vi "Test - copia (2).vi"() -> ()   [LabVIEW 2010]
panel:
  in  "Vi to open":enum16{"JILTest", "JILTest2", "JILTestR"}(ring)
  in  "stringin":string
  in  "booleanin":bool=TRUE
  in  "doublein":dbl
  in  "intin":i32
  in  "Mensajes":T1(ring)
  in  "stop":bool
  in  "Send":bool=TRUE
  out "error out":errorcluster
  out "Respuesta":string
  out "Mensaje":string
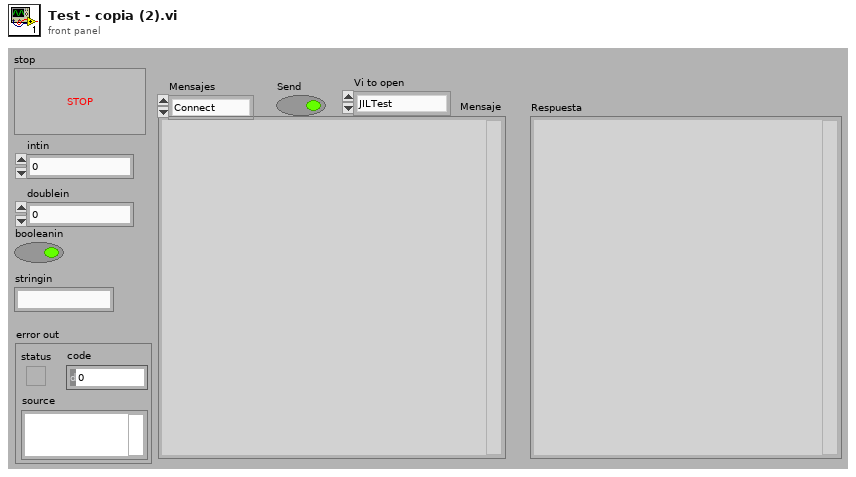
[diagram p1: front panel]
types:
  T1 = enum16{"Connect", "OpenVi", "SyncVi", "RunVi", "StopVi", "CloseVi", "Disconnect"}
  T2 = enum16{"Standard", "Buffered", "CRLF", "Immediate"}
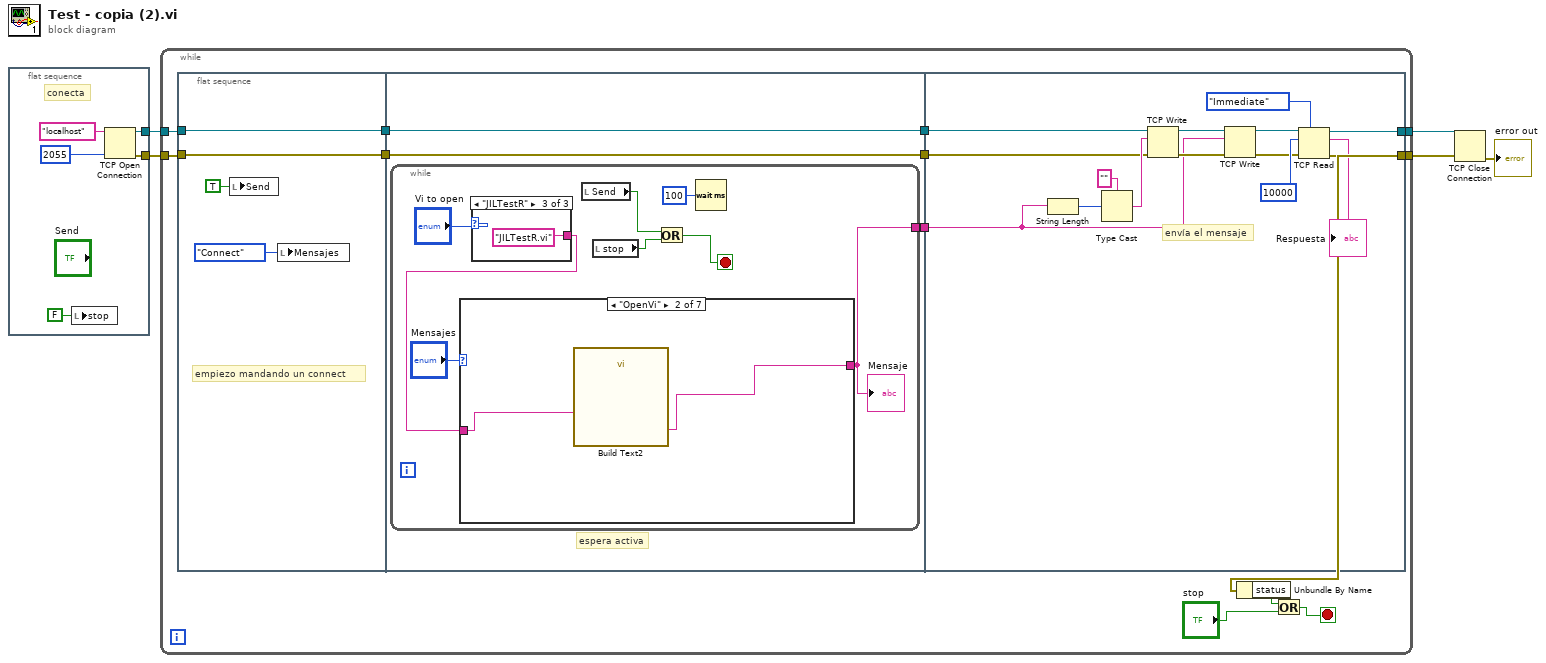
[diagram p0: block diagram]
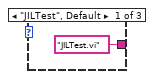
[diagram p2: hidden frame]
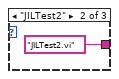
[diagram p3: hidden frame]
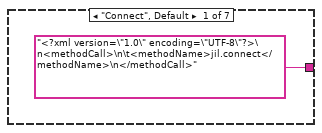
[diagram p4: hidden frame]
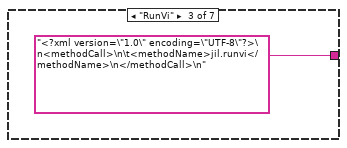
[diagram p5: hidden frame]
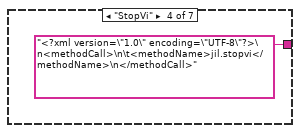
[diagram p6: hidden frame]
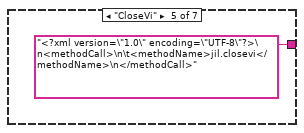
[diagram p7: hidden frame]
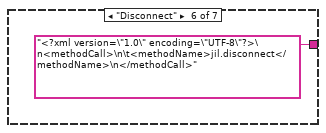
[diagram p8: hidden frame]
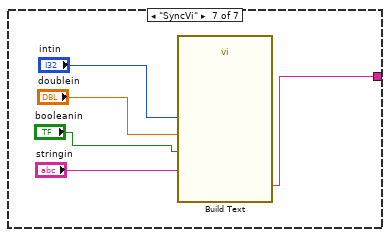
[diagram p9: hidden frame]
diagram:
  n1 = flat-sequence {
    tunnel: [w8] -> w5
    tunnel: [w7] -> w4
    frame #0 {
      # "conecta"
      n2 = local write "stop"(FALSE ("stop")) -> ()
      n3 = TCP Open Connection(address="localhost", remote port or service name=u16 2055) -> (connection ID=w8:refnum<k5>, error out=w7:errorcluster)  [unwired: 3 in]
    }
  }
  n4 = while {
    tunnel: w5 -> [w18]
    tunnel: w4 -> [w17]
    tunnel: [w16] -> w2
    tunnel: [w13] -> w1
    stop <- w14 stop-if-true
    n5 = flat-sequence {
      tunnel: w17 -> [w25]
      tunnel: [w25] -> w22
      tunnel: w18 -> [w24]
      tunnel: [w24] -> w21
      tunnel: w22 -> [w29]
      tunnel: [w29] -> w20
      tunnel: w21 -> [w28]
      tunnel: [w28] -> w19
      tunnel: [w27] -> w11
      tunnel: [w58] -> w16
      tunnel: [w57] -> w13
      tunnel: w20 -> [w56]
      tunnel: w19 -> [w55]
      tunnel: w11 -> [w53]
      frame #0 {
        # "empiezo mandando un connect"
        n6 = local write "Send"(TRUE ("Send")) -> ()
        n7 = local write "Mensajes"(T1."Connect" ("Mensajes")) -> ()
      }
      frame #1 {
        # "espera activa"
        n8 = while {
          tunnel: [w32] -> w27
          stop <- w36 stop-if-true
          n9 = case shown="\"JILTestR\"" "Vi to open" {
            tunnel: ["JILTest.vi" "JILTest2.vi" "JILTestR.vi"] -> w30
            frame "JILTest", Default {
            }
            frame "JILTest2" {
            }
            frame "JILTestR" {
            }
          }
          n10 = case shown="\"OpenVi\"" "Mensajes" {
            tunnel: ["<?xml version=\"1.0\" encoding=\"UTF-8\"?>\n<methodCall>\n\t<methodName>jil.connect</methodName>\n</methodCall>" w42 "<?xml version=\"1.0\" encoding=\"UTF-8\"?>\n<methodCall>\n\t<methodName>jil.runvi</methodName>\n</methodCall>\n" "<?xml version=\"1.0\" encoding=\"UTF-8\"?>\n<methodCall>\n\t<methodName>jil.stopvi</methodName>\n</methodCall>" "<?xml version=\"1.0\" encoding=\"UTF-8\"?>\n<methodCall>\n\t<methodName>jil.closevi</methodName>\n</methodCall>" "<?xml version=\"1.0\" encoding=\"UTF-8\"?>\n<methodCall>\n\t<methodName>jil.disconnect</methodName>\n</methodCall>" w52] -> w32
            tunnel: w30 -> [_ w43 _ _ _ _ _]
            frame "Connect", Default {
            }
            frame "OpenVi" {
              n11 = call "Build Text2"("name"=w43) -> ("Result"=w42:string)  [unwired: 13 in, 1 out]
            }
            frame "RunVi" {
            }
            frame "StopVi" {
            }
            frame "CloseVi" {
            }
            frame "Disconnect" {
            }
            frame "SyncVi" {
              n12 = call "Build Text"("string"="stringin", "int"="intin", "double"="doublein", "bolean"="booleanin") -> ("Result"=w52:string)  [unwired: 10 in, 1 out]
            }
          }
          "Mensaje" <- w32
          n13 = local read "Send"() -> (w34:bool)
          n14 = local read "stop"() -> (w35:bool)
          n15 = Or(x=w34, y=w35) -> (x .or. y?=w36:bool)
          n16 = Wait (ms)(milliseconds to wait=u32 100) -> ()  [unwired: 1 out]
        }
      }
      frame #2 {
        # "envía el mensaje"
        n17 = String Length(string=w53) -> (length=w61:i32)
        n18 = Type Cast(type="", x=w61) -> (*(type *) &x=w63:string)
        n19 = TCP Write(connection ID=w55, data in=w63, error in (no error)=w56) -> (connection ID out=w59:refnum<k5>, error out=w60:errorcluster)  [unwired: 1 in, 1 out]
        n20 = TCP Write(connection ID=w59, data in=w53, error in (no error)=w60) -> (connection ID out=w64:refnum<k5>, error out=w65:errorcluster)  [unwired: 1 in, 1 out]
        n21 = TCP Read(connection ID=w64, bytes to read=10000, error in (no error)=w65, 7:T2."Immediate" ("mode (standard)")) -> (connection ID out=w58:refnum<k5>, data out=→"Respuesta":string, error out=w57:errorcluster)  [unwired: 1 in]
      }
    }
    n22 = Unbundle By Name(w13) -> ("status"=w12:bool)
    n23 = Or(x=w12, y="stop") -> (x .or. y?=w14:bool)
  }
  n24 = TCP Close Connection(connection ID=w2, error in (no error)=w1) -> (error out=→"error out":errorcluster)  [unwired: 1 in, 1 out]
